vi "Load Image.vi"(8 "error in (no error)":errorcluster, 10 "path to PNG file":path=path "C:/Users/jhobson/Desktop/logo.png", 11 "Picture Ref":refnum<vi>) -> (0 "error out":errorcluster)   [LabVIEW 2020]
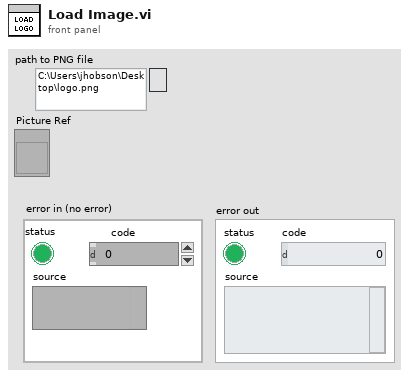
[diagram p1: front panel]
types:
  T1 = typedef "imagedata.ctl" = cluster{"image type":i32, "image depth":i32, "image":u8[], "mask":u8[], "colors":u32[], "Rectangle":cluster{"left":i16, "top":i16, "right":i16, "bottom":i16}}
  T2 = typedef "LVBoundsTypeDef.ctl" = cluster{"Width":u32, "Height":u32}
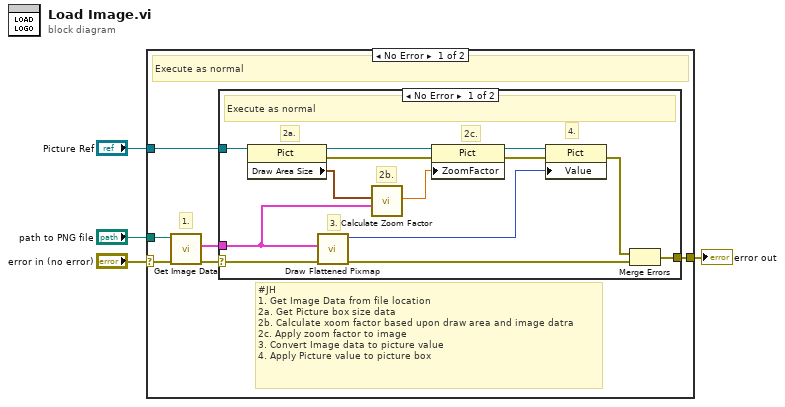
[diagram p0: block diagram]
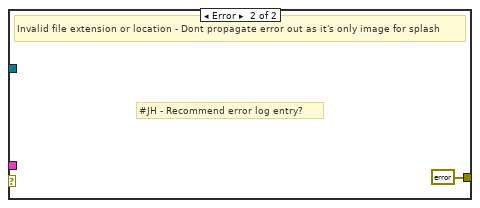
[diagram p2: hidden frame]
diagram:
  n1 = case shown="No Error" "error in (no error)" {
    selector: "error in (no error)" -> [w6 w24]
    tunnel: "Picture Ref" -> [w10 _]
    tunnel: [w8 w24] -> w3
    tunnel: "path to PNG file" -> [w7 _]
    frame No Error {
      # "#JH\n1. Get Image Data from file location\n2a. Get Picture box size data\n2b. Calculate xoom factor based upon draw area and image datra\n2c. Apply zoom factor to image\n3. Convert Image data to picture value\n4. Apply Picture value to picture box"
      # "1."
      # "Execute as normal"
      n2 = call "Get Image Data.vi"("error in (no error)"=w6, "path to PNG file"=w7) -> ("error out"=w9:errorcluster, "image data"=w5:T1)  [unwired: 8 in]
      n3 = case shown="No Error" w9 {
        selector: w9 -> [w15 _]
        tunnel: w10 -> [w22 _]
        tunnel: [w14 errorcluster {"status"=FALSE, "code"=0, "source"=""} ("error IO")] -> w8
        tunnel: w5 -> [w13 _]
        frame No Error {
          # "4."
          # "2c."
          # "2a."
          # "2b."
          # "3."
          # "Execute as normal"
          n4 = property class="Pict"(reference=w22) -> (reference out=w21:refnum<vi>, error out=w18:errorcluster, "Draw Area Size"=w12:T2)  [unwired: 1 in]
          n5 = call <vilib>:"Draw Flattened Pixmap.vi"("image data"=w13) -> ("new picture"=w20:picture)  [unwired: 8 in]
          n6 = call "Calculate Zoom Factor.vi"("image data"=w13, "Draw Area Size"=w12) -> ("Zoom Factor"=w11:dbl)  [unwired: 9 in]
          n7 = property class="Pict"(reference=w21, error in=w18, "ZoomFactor"=w11) -> (reference out=w19:refnum<vi>, error out=w17:errorcluster)
          n8 = property class="Pict"(reference=w19, error in=w17, "Value"=w20) -> (error out=w16:errorcluster)  [unwired: 1 out]
          n9 = Merge Errors(w16, w15) -> (w14:errorcluster)
        }
        frame Error {
          # "#JH - Recommend error log entry?"
          # "Invalid file extension or location - Dont propagate error out as it's only image for splash"
        }
      }
    }
    frame Error {
      # "Error Propagated In - Do Nothing"
    }
  }
  "error out" <- w3
